vi "Check alarms.vi"(0 "alarms":T1, 11 "error in (no error)":errorcluster) -> (15 "error out":errorcluster)   [LabVIEW 2019]
uses:
  <instrlib>/niMmWave/ni3610 and ni3630/controls/public/DAC Alarms.ctl
  <instrlib>/niMmWave/ni3610 and ni3630/ni3610_and_ni3630_Driver_Lib.lvlib
panel:
  # "Lane Number"
  # "0     1     2    3     4    5     6    7"
  # "Multiframe Alignment Error"
  # "Frame Alignment Error"
  # "Link Configuration Error"
  # "Elastic Buffer Overflow"
  # "Elastic Buffer Match Error"
  # "Code Group Synch. Error"
  # "8b/10b Not-in-Table Error"
  # "8b/10b Disparity Error"
  # "Lane Number"
  # "0     1     2    3     4    5     6    7"
  # "FIFO Write Error"
  # "FIFO Write Full"
  # "FIFO Read Error"
  # "FIFO Read Empty"
  # "Short Test Error"
  # "LOS Detect Alarm"
  # "SYSREF Alarms\n0      1      2     3"
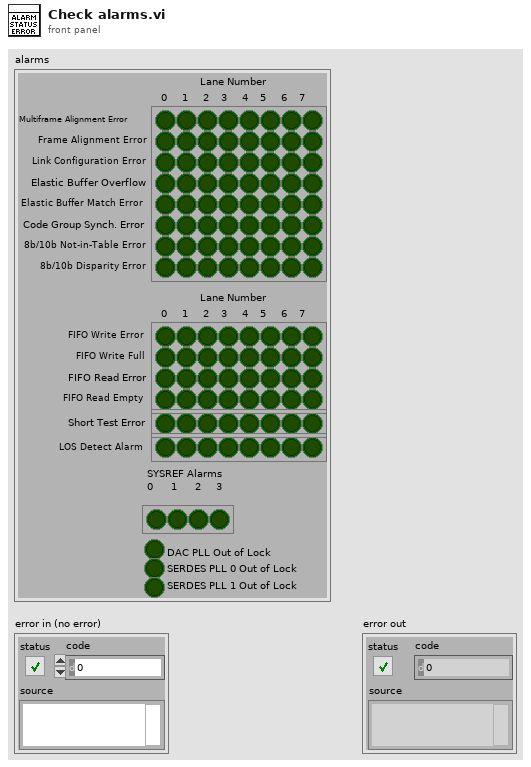
[diagram p1: front panel]
types:
  T1 = typedef "ni3610_and_ni3630_Driver_Lib.lvlib/DAC Alarms.ctl" = cluster{"Lane Errors":bool[][], "FIFO Errors":bool[][], "Short Test Alarms":bool[], "LOS Alarms":bool[], "SYSREF Errors":bool[], "DAC38J84 PLL Out of Lock 3":bool, "DAC38J84 RW0 Out of Lock 3":bool, "DAC38J84 RW1 Out of Lock 3":bool}
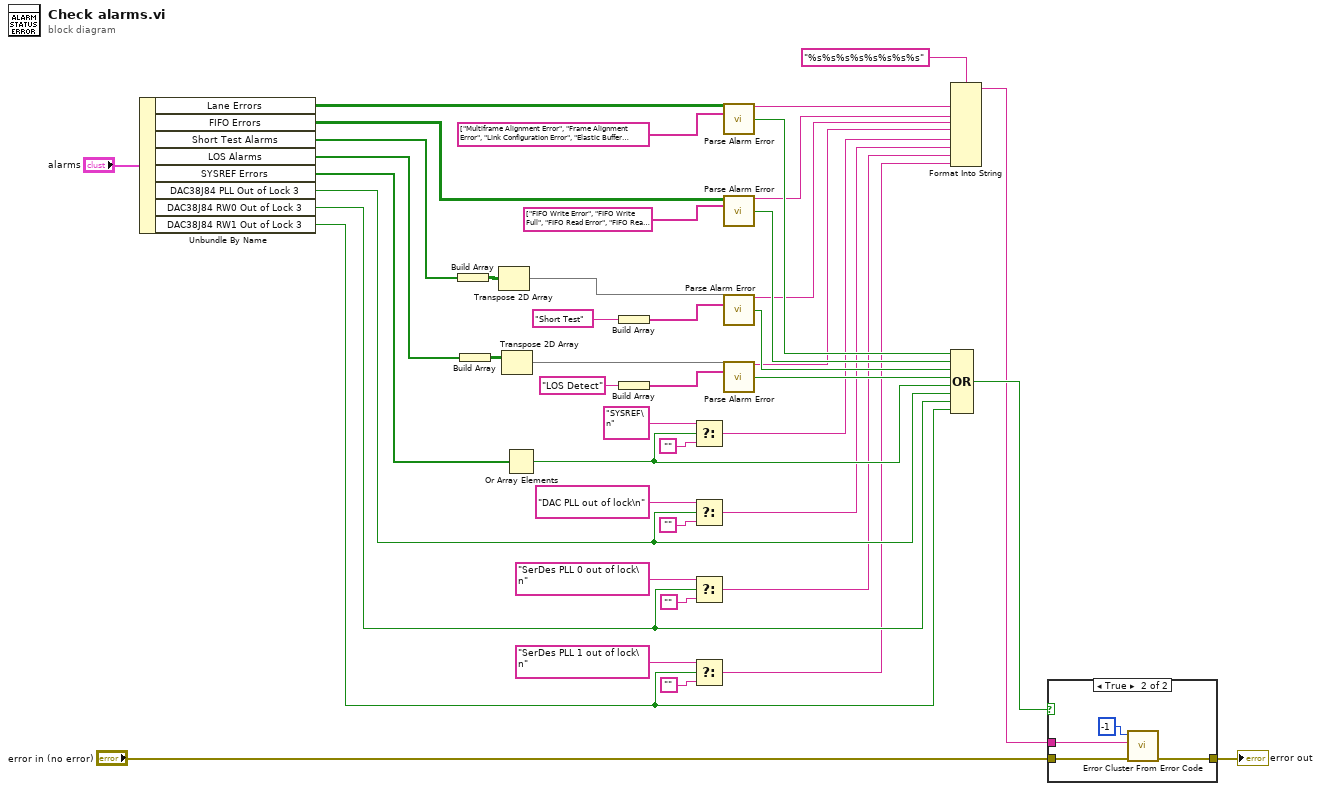
[diagram p0: block diagram]
diagram:
  n1 = Unbundle By Name("alarms") -> ("Lane Errors"=w31:bool[][], "FIFO Errors"=w32:bool[][], "Short Test Alarms"=w40:bool[], "LOS Alarms"=w44:bool[], "SYSREF Errors"=w21:bool[], "DAC38J84 PLL Out of Lock 3"=w11:bool, "DAC38J84 RW0 Out of Lock 3"=w10:bool, "DAC38J84 RW1 Out of Lock 3"=w9:bool)
  n2 = Build Array(w40) -> (w39:bool[][])
  n3 = Build Array(w44) -> (w38:bool[][])
  n4 = Transpose 2D Array(2D array=w39) -> (transposed array=w34:bool[][])
  n5 = Transpose 2D Array(2D array=w38) -> (transposed array=w33:bool[][])
  n6 = Or Array Elements(Boolean array=w21) -> (logical OR=w20:bool)
  n7 = Build Array("Short Test") -> (w36:string[])
  n8 = Build Array("LOS Detect") -> (w35:string[])
  n9 = Select(t="SYSREF\n", s=w20, f="") -> (s? t:f=w8:string)
  n10 = Select(t="DAC PLL out of lock\n", s=w11, f="") -> (s? t:f=w7:string)
  n11 = Select(t="SerDes PLL 0 out of lock\n", s=w10, f="") -> (s? t:f=w6:string)
  n12 = Select(t="SerDes PLL 1 out of lock\n", s=w9, f="") -> (s? t:f=w5:string)
  n13 = call "Parse Alarm Error.vi"("errors"=w31, "error description"=string[] ["Multiframe Alignment Error", "Frame Alignment Error", "Link Configuration Error", "Elastic Buffer Overflow", "Elastic Buffer Match Error", "Code Group Synch. Error", "8b/10b Not-in-Table Error", "8b/10b Disparity Error"] ("Lane Errors")) -> ("error description"=w26:string, "error"=w30:bool)  [unwired: 12 in]
  n14 = call "Parse Alarm Error.vi"("errors"=w32, "error description"=string[] ["FIFO Write Error", "FIFO Write Full", "FIFO Read Error", "FIFO Read Empty"] ("FIFO Errors")) -> ("error description"=w24:string, "error"=w29:bool)  [unwired: 12 in]
  n15 = call "Parse Alarm Error.vi"("errors"=w34, "error description"=w36) -> ("error description"=w23:string, "error"=w28:bool)  [unwired: 12 in]
  n16 = call "Parse Alarm Error.vi"("errors"=w33, "error description"=w35) -> ("error description"=w22:string, "error"=w27:bool)  [unwired: 12 in]
  n17 = Format Into String(format string="%s%s%s%s%s%s%s%s", w26, w24, w23, w22, w8, w7, w6, w5) -> (resulting string=w1:string)  [unwired: 2 in, 1 out]
  n18 = Compound Arithmetic op=OR(w30, w29, w28, w27, w20, w11, w10, w9) -> (w2:bool)
  n19 = case shown="True" w2 {
    tunnel: "error in (no error)" -> [w46 w50]
    tunnel: [w46 w49] -> w3
    tunnel: w1 -> [_ w48]
    frame False {
    }
    frame True {
      n20 = call <vilib>:"Error Cluster From Error Code.vi"("error in (no error)"=w50, "error message (\"\")"=w48, "error code (0)"=-1) -> ("error out"=w49:errorcluster)  [unwired: 6 in]
    }
  }
  "error out" <- w3
